vi "Move to Hallway.vi"(8 "Max Score":i64=60000, 11 "Data In":T1) -> (3 "Data Out":T1[](array[typedef]))   [LabVIEW 2020]
uses:
  Data.ctl
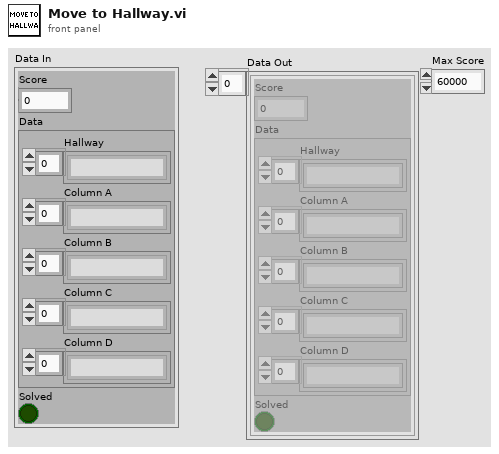
[diagram p1: front panel]
types:
  T1 = typedef "Data.ctl" = cluster{"Score":i64, "Data":cluster{"Hallway":string[], "Column A":string[], "Column B":string[], "Column C":string[], "Column D":string[]}, "Solved":bool}
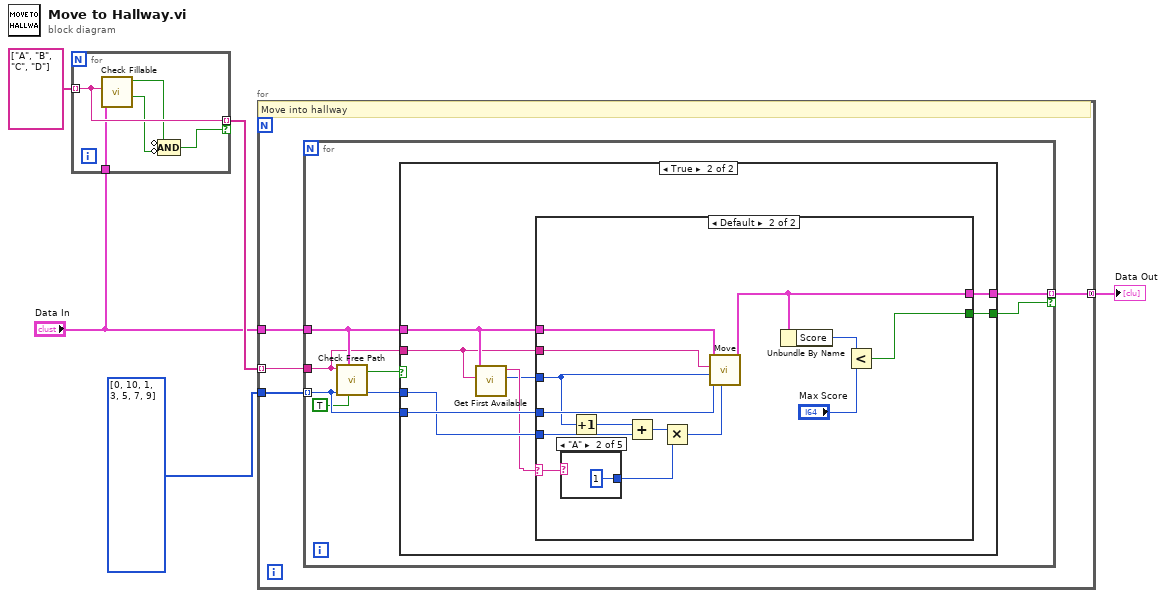
[diagram p0: block diagram]
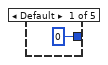
[diagram p4: hidden frame]
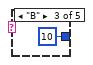
[diagram p5: hidden frame]
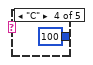
[diagram p6: hidden frame]
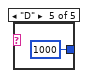
[diagram p7: hidden frame]
diagram:
  n1 = for {
    tunnel: string[] ["A", "B", "C", "D"] -> [w10] mode=indexing
    tunnel: [w10] -> w4 mode=indexing if=w6
    tunnel: "Data In" -> [w9]
    n2 = call "Check Fillable.vi"("Column"=w10, "Data In"=w9) -> ("Full?"=w7:bool, "Fillable"=w8:bool)  [unwired: 7 in, 1 out]
    n3 = Compound Arithmetic op=AND(invert w8, invert w7) -> (w6:bool)
  }
  n4 = for {
    tunnel: "Data In" -> [w13]
    tunnel: i32[] [0, 10, 1, 3, 5, 7, 9] ("indices") -> [w14]
    tunnel: w4 -> [w12] mode=indexing
    tunnel: [w11] -> w1 mode=concatenating
    # "Move into hallway"
    n5 = for {
      tunnel: w14 -> [w21] mode=indexing
      tunnel: w13 -> [w20]
      tunnel: w12 -> [w18]
      tunnel: [w16] -> w11 mode=indexing if=w15
      n6 = call "Check Free Path.vi"("To Hallway"=TRUE, "Data In"=w20, "Hallway Index"=w21, "Column"=w18) -> ("Length"=w19:i32, "Free Path?"=w22:bool)  [unwired: 6 in]
      n7 = case shown="True" w22 {
        tunnel: w21 -> [_ w30]
        tunnel: w20 -> [_ w28]
        tunnel: w19 -> [_ w29]
        tunnel: w18 -> [_ w25]
        tunnel: [_ w24] -> w16
        tunnel: [_ w23] -> w15
        frame False {
        }
        frame True {
          n8 = call "Get First Available.vi"("Column"=w25, "Data In"=w28) -> ("Index"=w26:i64, "Value"=w27:string)  [unwired: 8 in]
          n9 = case shown="Default" w27 {
            selector: w27 -> [_ w38]
            tunnel: w30 -> [_ w44]
            tunnel: w28 -> [_ w41]
            tunnel: w29 -> [_ w40]
            tunnel: w25 -> [_ w36]
            tunnel: w26 -> [_ w37]
            tunnel: [_ w34] -> w24
            tunnel: [_ w31] -> w23
            frame "." {
            }
            frame Default {
              n10 = case shown="\"A\"" w38 {
                tunnel: [i64 0 i64 1 i64 10 i64 100 i64 1000] -> w42
                frame Default {
                }
                frame "A" {
                }
                frame "B" {
                }
                frame "C" {
                }
                frame "D" {
                }
              }
              n11 = Increment(x=w37) -> (x+1=w39:i64)
              n12 = Add(x=w39, y=w40) -> (x+y=w43:i64)
              n13 = Multiply(x=w43, y=w42) -> (x*y=w35:i64)
              n14 = call "Move.vi"("Cost"=w35, "Hallway Index"=w44, "Column Index"=w37, "Column"=w36, "Data In"=w41) -> ("Data Out"=w34:T1)  [unwired: 6 in]
              n15 = Unbundle By Name(w34) -> ("Score"=w33:i64)
              n16 = Less?(x=w33, y="Max Score") -> (x < y?=w31:bool)
            }
          }
        }
      }
    }
  }
  "Data Out" <- w1
